vi "Read Modified Time.vi"(8 "Error In":errorcluster) -> (0 "Error Out":errorcluster)   [LabVIEW 2018, in "Tests.lvlib" / "File Info.lvlib"]
uses:
  File Info.lvlib
  src/Toolkit/File Info/File Info.lvclass/File Info.ctl
  src/Toolkit/SSH/SSH.lvclass/SSH.ctl
  src/Toolkit/SSH/Utility/Read Shared Library.vi
  src/Toolkit/Support/Check Status.vi
  <vilib>/addons/_JKI Toolkits/Caraya/classes/Test/Test.lvclass
  <vilib>/addons/_JKI Toolkits/Caraya/classes/Assert/Assert.lvclass
  src/Toolkit/File Info/File Info.lvclass
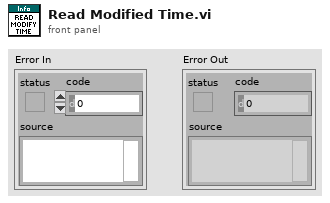
[diagram p1: front panel]
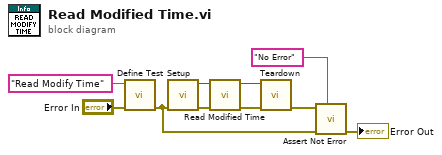
[diagram p0: block diagram]
diagram:
  n1 = call <vilib>:"Define Test.vi"("error in (no error)"="Error In", "Label (VI Title)"="Read Modify Time") -> ("error out"=w6:errorcluster)  [unwired: 9 in]
  n2 = call "Setup.vi"("Error In"=w6) -> ("Error Out"=w3:errorcluster, "File Info"=w4:refnum<class "File Info.lvclass">)  [unwired: 9 in]
  n3 = call "Read Modified Time.vi"("Error In"=w3, "File Info In"=w4) -> ("Error Out"=w1:errorcluster, "File Info Out"=w2:refnum<class "File Info.lvclass">)  [unwired: 7 in, 1 out]
  n4 = call "Teardown.vi"("Error In"=w1, "File Info"=w2) -> ("Error Out"=w5:errorcluster)  [unwired: 9 in]
  n5 = call <vilib>:"Assert Not Error.vi"("Label"="No Error", "error in (no error)"=w6, "Not Error?"=w5) -> ("error out"=→"Error Out":errorcluster)  [unwired: 8 in]
